vi "Divide signals.vi"(0 "All data":waveform(dbl)[](array[waveform])) -> (1 "Voltages":waveform(dbl)[](array[waveform]), 2 "Currents":waveform(dbl)[](array[waveform]))   [LabVIEW 2020]
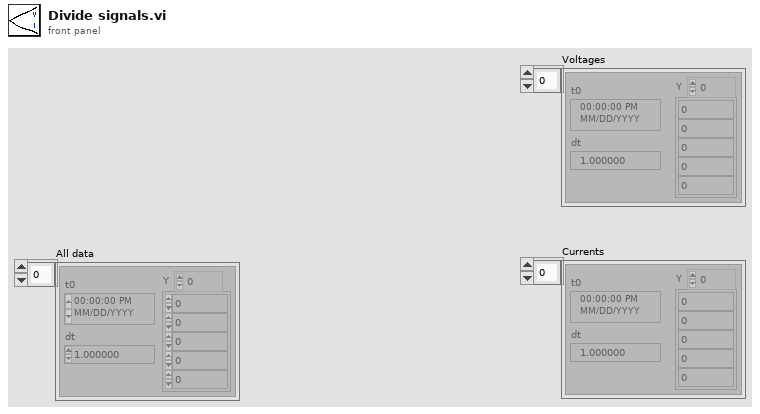
[diagram p1: front panel]
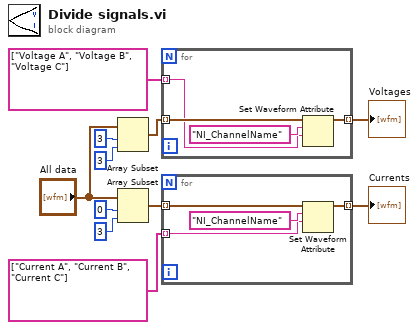
[diagram p0: block diagram]
diagram:
  n1 = Array Subset(array="All data", index=3, length=3) -> (w2:waveform(dbl)[])
  n2 = Array Subset(array="All data", index=0, length=3) -> (w6:waveform(dbl)[])
  n3 = for {
    tunnel: w2 -> [w15] mode=indexing
    tunnel: string[] ["Voltage A", "Voltage B", "Voltage C"] -> [w13] mode=indexing
    tunnel: [w12] -> w3 mode=indexing
    n4 = Set Waveform Attribute(5:w13, 6:"NI_ChannelName" ("name"), 7:w15) -> (3:w12:waveform(dbl))  [unwired: 1 in, 2 out]
  }
  "Voltages" <- w3
  n5 = for {
    tunnel: w6 -> [w19] mode=indexing
    tunnel: string[] ["Current A", "Current B", "Current C"] -> [w17] mode=indexing
    tunnel: [w16] -> w4 mode=indexing
    n6 = Set Waveform Attribute(5:w17, 6:"NI_ChannelName" ("name"), 7:w19) -> (3:w16:waveform(dbl))  [unwired: 1 in, 2 out]
  }
  "Currents" <- w4
